vi "report data.vi"() -> (0 "Model Selection":i32, 1 "VW_ Medium":T1, 3 "SK Global":T1, 6 "Data":string[](array[string]))   [LabVIEW 2015]
uses:
  <vilib>/Utility/error.llb/whitespace.ctl
  Galobal variable_TI.vi
panel:
  out "size(s) 4":i32
  out "size(s) 3":i32
  out "size(s) 2":i32
  out "size(s)":i32
  out "date/time string":string
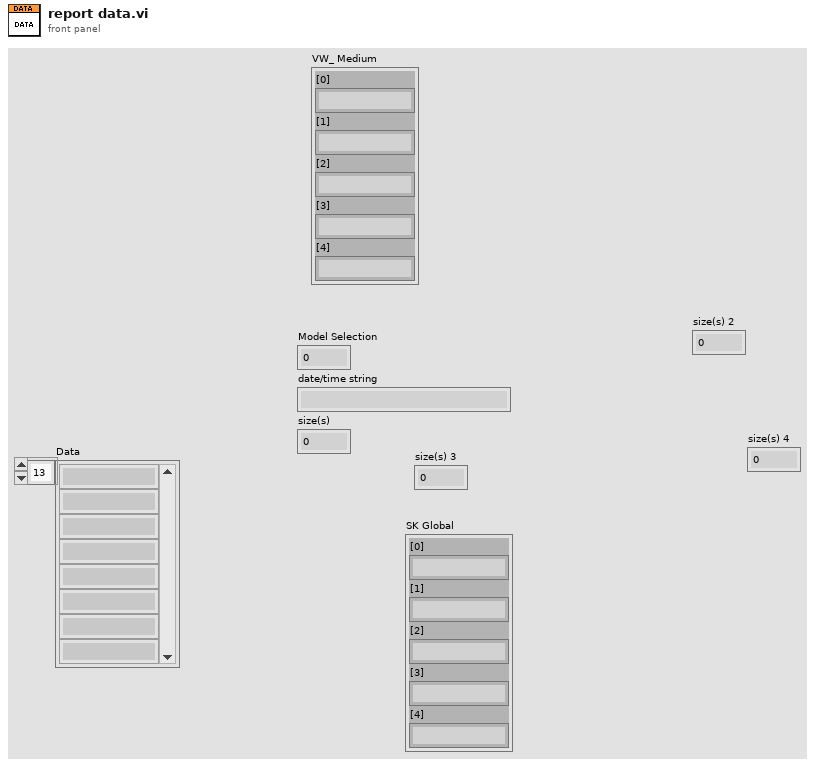
[diagram p1: front panel]
types:
  T1 = cluster{"[0]":string, "[1]":string, "[2]":string, "[3]":string, "[4]":string}
  T2 = typedef "whitespace.ctl" = u16
  T3 = cluster{"MaxLoad ":dbl, "Min Load":dbl, "MaxDistance(mm)":dbl, "Min Distance(mm)":dbl, "Load Offset":dbl, "Model":string, "Difusser Code":string, "TFT Code ":string, "LVDT Offset":dbl}
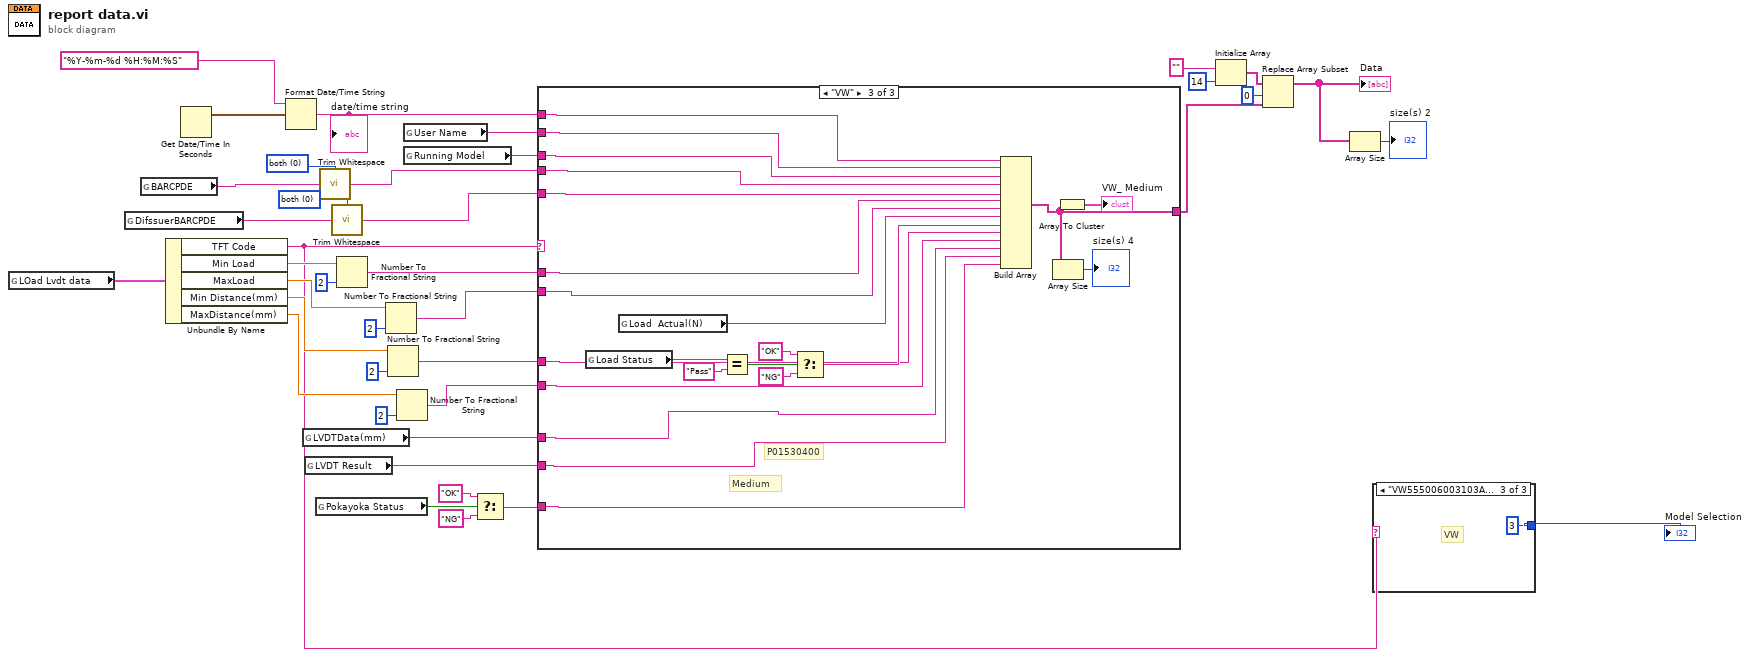
[diagram p0: block diagram]
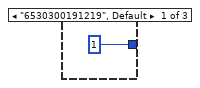
[diagram p2: hidden frame]
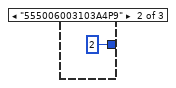
[diagram p3: hidden frame]
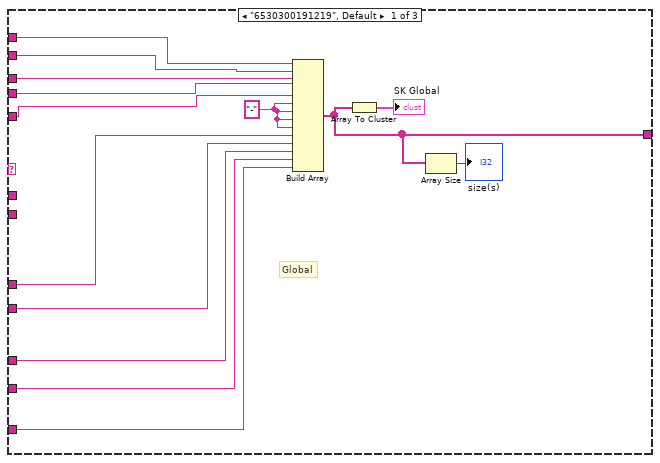
[diagram p4: hidden frame]
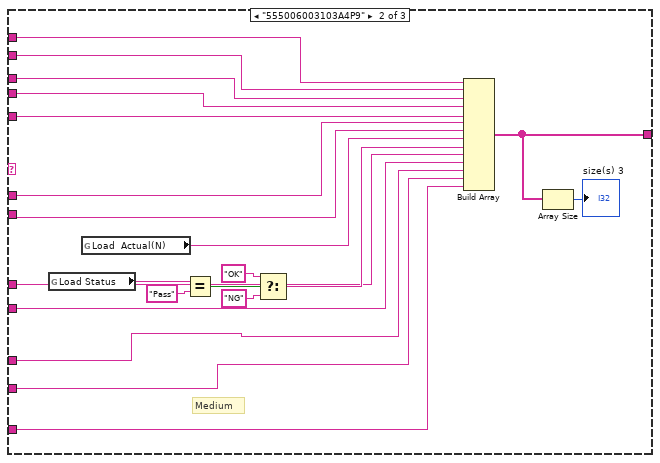
[diagram p5: hidden frame]
diagram:
  w10 = T2 0 items=["both", "start of string", "end of string"] ("location (both)")
  w13 = T2 0 items=["both", "start of string", "end of string"] ("location (both)")
  n1 = global read "Galobal variable_TI.vi" "LOad Lvdt data"() -> (w39:T3)
  n2 = global read "Galobal variable_TI.vi" "DifssuerBARCPDE"() -> (w9:string)
  n3 = global read "Galobal variable_TI.vi" "BARCPDE"() -> (w12:string)
  n4 = Unbundle By Name(w39) -> ("TFT Code"=w15:string, "Min Load"=w38:dbl, "MaxLoad"=w33:dbl, "Min Distance(mm)"=w32:dbl, "MaxDistance(mm)"=w31:dbl)
  n5 = Get Date/Time In Seconds() -> (seconds since 1Jan1904=w20:timestamp)
  n6 = Format Date/Time String(time format string (%c)="%Y-%m-%d %H:%M:%S", seconds (now)=w20) -> (date/time string=w19:string)  [unwired: 1 in]
  "date/time string" <- w19
  n7 = global read "Galobal variable_TI.vi" "LVDTData(mm)"() -> (w16:string)
  n8 = global read "Galobal variable_TI.vi" "LVDT Result"() -> (w17:string)
  n9 = global read "Galobal variable_TI.vi" "Pokayoka Status"() -> (w24:bool)
  n10 = call <vilib>:"Trim Whitespace.vi"("string"=w12, "location (both)"=w13) -> ("trimmed string"=w11:string)
  n11 = call <vilib>:"Trim Whitespace.vi"("string"=w9, "location (both)"=w10) -> ("trimmed string"=w8:string)
  n12 = Number To Fractional String(number=w38, precision (6)=i16 2) -> (F-format string=w30:string)  [unwired: 2 in]
  n13 = Number To Fractional String(number=w33, precision (6)=i16 2) -> (F-format string=w29:string)  [unwired: 2 in]
  n14 = Number To Fractional String(number=w32, precision (6)=i16 2) -> (F-format string=w28:string)  [unwired: 2 in]
  n15 = Number To Fractional String(number=w31, precision (6)=i16 2) -> (F-format string=w27:string)  [unwired: 2 in]
  n16 = global read "Galobal variable_TI.vi" "User Name"() -> (w22:string)
  n17 = global read "Galobal variable_TI.vi" "Running Model"() -> (w21:string)
  n18 = Select(t="OK", s=w24, f="NG") -> (s? t:f=w23:string)
  n19 = case shown="\"VW\"" w15 {
    tunnel: w30 -> [_ w74 w83]
    tunnel: w29 -> [_ w73 w82]
    tunnel: w28 -> [w43 w65 w81]
    tunnel: w27 -> [w44 w64 w80]
    tunnel: w23 -> [w47 w63 w77]
    tunnel: w22 -> [w52 w62 w87]
    tunnel: w21 -> [w51 w61 w86]
    tunnel: w11 -> [w50 w60 w85]
    tunnel: w8 -> [w49 w59 w84]
    tunnel: w19 -> [w53 w58 w88]
    tunnel: w17 -> [w46 w56 w78]
    tunnel: w16 -> [w45 w57 w79]
    tunnel: [w41 w54 w75] -> w3
    frame "6530300191219", Default {
      w42 = "-" ("element")
      # "Global"
      n20 = Build Array(w53, w52, w51, w50, w49, w42, w42, w42, w42, w43, w44, w45, w46, w47) -> (w41:string[])
      n21 = Array To Cluster(array=w41) -> (cluster=→"SK Global":T1)
      n22 = Array Size(array=w41) -> (size(s)=→"size(s)":i32)
    }
    frame "555006003103A4P9" {
      # "Medium"
      n23 = global read "Galobal variable_TI.vi" "Load Status"() -> (w71:string)
      n24 = global read "Galobal variable_TI.vi" "Load  Actual(N)"() -> (w72:string)
      n25 = Equal?(x=w71, y="Pass") -> (x = y?=w69:bool)
      n26 = Select(t="OK", s=w69, f="NG") -> (s? t:f=w66:string)
      n27 = Build Array(w58, w62, w61, w60, w59, w74, w73, w72, w66, w65, w64, w57, w56, w63) -> (w54:string[])
      n28 = Array Size(array=w54) -> (size(s)=→"size(s) 3":i32)
    }
    frame "VW" {
      # "Medium"
      # "P01530400"
      n29 = global read "Galobal variable_TI.vi" "Load Status"() -> (w95:string)
      n30 = global read "Galobal variable_TI.vi" "Load  Actual(N)"() -> (w96:string)
      n31 = Equal?(x=w95, y="Pass") -> (x = y?=w93:bool)
      n32 = Select(t="OK", s=w93, f="NG") -> (s? t:f=w90:string)
      n33 = Build Array(w88, w87, w86, w85, w84, w83, w82, w96, w90, w81, w80, w79, w78, w77) -> (w75:string[])
      n34 = Array Size(array=w75) -> (size(s)=→"size(s) 4":i32)
      n35 = Array To Cluster(array=w75) -> (cluster=→"VW_ Medium":T1)
    }
  }
  n36 = Initialize Array("", 14 ("dimension size")) -> (w6:string[])
  n37 = Replace Array Subset(array=w6, new element=w3, index=0) -> (w1:string[])
  "Data" <- w1
  n38 = Array Size(array=w1) -> (size(s)=→"size(s) 2":i32)
  n39 = case shown="\"VW555006003103A4P9\"" w15 {
    tunnel: [1 2 3] -> w14
    frame "6530300191219", Default {
    }
    frame "555006003103A4P9" {
    }
    frame "VW555006003103A4P9" {
      # "VW"
    }
  }
  "Model Selection" <- w14
